vi "Read Results from processing.vi"(8 "error in":errorcluster, 11 "fixed channel tag bus module in":refnum<class "fixed channel tag bus module.lvclass">) -> (0 "error out":errorcluster, 2 "Results from processing":T1, 3 "fixed channel tag bus module out":refnum<class "fixed channel tag bus module.lvclass">)   [LabVIEW 2013, in "fixed channel tag bus module.lvclass"]
uses:
  fixed channel tag bus module.lvclass
  Runtime data typedefs/results.ctl
  fixed channel tag bus module.lvclass/fixed channel tag bus module.ctl
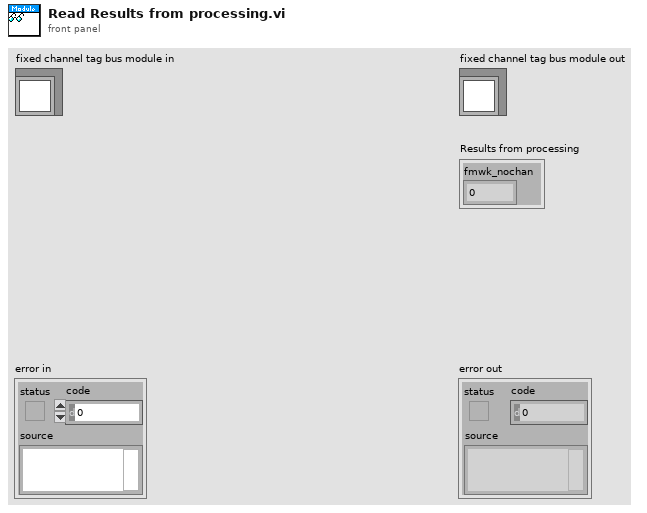
[diagram p1: front panel]
types:
  T1 = typedef "fixed channel tag bus module.lvclass/results.ctl" = cluster{"fmwk_nochan":i32}
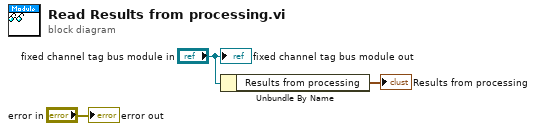
[diagram p0: block diagram]
diagram:
  n1 = Unbundle By Name("fixed channel tag bus module in") -> ("Results from processing"=→"Results from processing":T1)
  "error out" <- "error in"
  "fixed channel tag bus module out" <- "fixed channel tag bus module in"
